vi "2 Smooth controls.vi"(4 "Setpoints in":T1) -> (1 "Smoothed Setpoints out":T1)   [LabVIEW 2011]
doc: "Smooths rudder and sail setpoints. This is to avoid killing speed or wasting energy by moving controls too fast or too much.\nCurrently only smooths the rudder setpoint, but some kind of control (hysteretic?) for the sails could be implemented later.\nTODO: check that this actually helps, and see if there are ways to optimize it.\nTODO: remove smoothing for sails when the winch is more mechanically functional.\n-Jason"
uses:
  2 Typedefs/setpoints to boat.ctl
  2 Typedefs/sail setpt.ctl
  2 Typedefs/rudder angle.ctl
panel:
  in  "Maximum Sail Slew Rate (#/s)":dbl=0.1
  in  "Maximum Rudder Slew Rate (deg/s)":dbl=100.0
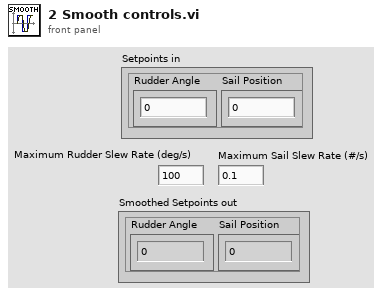
[diagram p1: front panel]
types:
  T1 = typedef "setpoints to boat.ctl" = cluster{"Sail Position":T2, "Rudder Angle":T3}
  T2 = typedef "sail setpt.ctl" = dbl
  T3 = typedef "rudder angle.ctl" = dbl
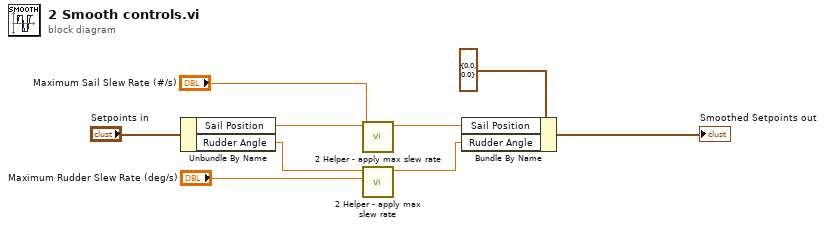
[diagram p0: block diagram]
diagram:
  n1 = Unbundle By Name("Setpoints in") -> ("Sail Position"=w2:T2, "Rudder Angle"=w7:T3)
  n2 = call "2 Helper - apply max slew rate.vi"("Maximum Slew Rate (#/s)"="Maximum Sail Slew Rate (#/s)", "Control Value In"=w2) -> ("Control Value Out"=w3:dbl)  [unwired: 9 in]
  n3 = call "2 Helper - apply max slew rate.vi"("Maximum Slew Rate (#/s)"="Maximum Rudder Slew Rate (deg/s)", "Control Value In"=w7) -> ("Control Value Out"=w6:dbl)  [unwired: 9 in]
  n4 = Bundle By Name(cluster=T1 {"Sail Position"=0.0, "Rudder Angle"=0.0} ("Final Setpoints 2"), "Sail Position"=w3, "Rudder Angle"=w6) -> (→"Smoothed Setpoints out":T1)
